vi "get acquisition timings - subvi.vi"(8 "error in (no error)":errorcluster, 9 "Kinetic Cycle Time (s)":dbl, 10 "Accumulation Cycle (s)":dbl, 11 "Exposure Time (sec)":sgl) -> (0 "error out":errorcluster, 1 "Kinetics":dbl format="%#_13g", 2 "Accumulation":dbl format="%#_13g", 3 "Exposure (s)":dbl format="%#_13g")   [LabVIEW 2014]
uses:
  Library Files - Andor and MadCity/Andorlib/atmcd32d.lvlib
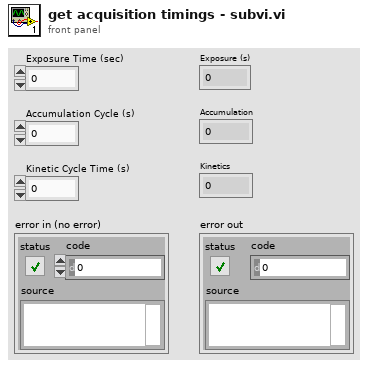
[diagram p1: front panel]
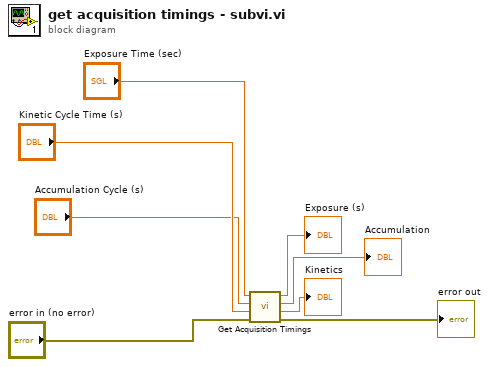
[diagram p0: block diagram]
diagram:
  n1 = call "Get Acquisition Timings.vi"("error in (no error)"="error in (no error)", "kinetic"="Kinetic Cycle Time (s)", "accumulate"="Accumulation Cycle (s)", "exposure"="Exposure Time (sec)") -> ("error out"=→"error out":errorcluster, "kinetic out"=→"Kinetics":sgl, "accumulate out"=→"Accumulation":sgl, "exposure out"=→"Exposure (s)":sgl)  [unwired: 3 in, 1 out]
